vi "Simulation Interface.vi"(8 "error in (no error)":errorcluster, 11 "View Model":T1) -> (0 "error out":errorcluster, 3 "View Model":T1)   [LabVIEW 2017]
doc: "Main VI used to validate the CarWash controller logic and algorithms."
uses:
  Model/Controls/View Model.ctl
  Model/Controls/Shared Model.ctl
  Error Handler/Controls/Error Model.ctl
  Error Handler/Controls/Error Message.ctl
  Error Handler/Controls/Error Type.ctl
  Configuration/Controls/Config Model.ctl
  Configuration/Controls/Config DB Message.ctl
  Configuration/Controls/Config DB Command.ctl
  Configuration/Controls/Config DB Overhead.ctl
  Configuration/Controls/Config DB Record1.ctl
  Configuration/Controls/Config DB Record2.ctl
  Controller/Controls/Controller Wash Step.ctl
  Views/Vehicle Position Simulation View/Controls/Vehicle - Position.ctl
  Controller/Controls/Controller Model.ctl
  Controller/Controls/Controller Overhead.ctl
  Controller/Controls/Controller State.ctl
  Model/Controls/Interface.ctl
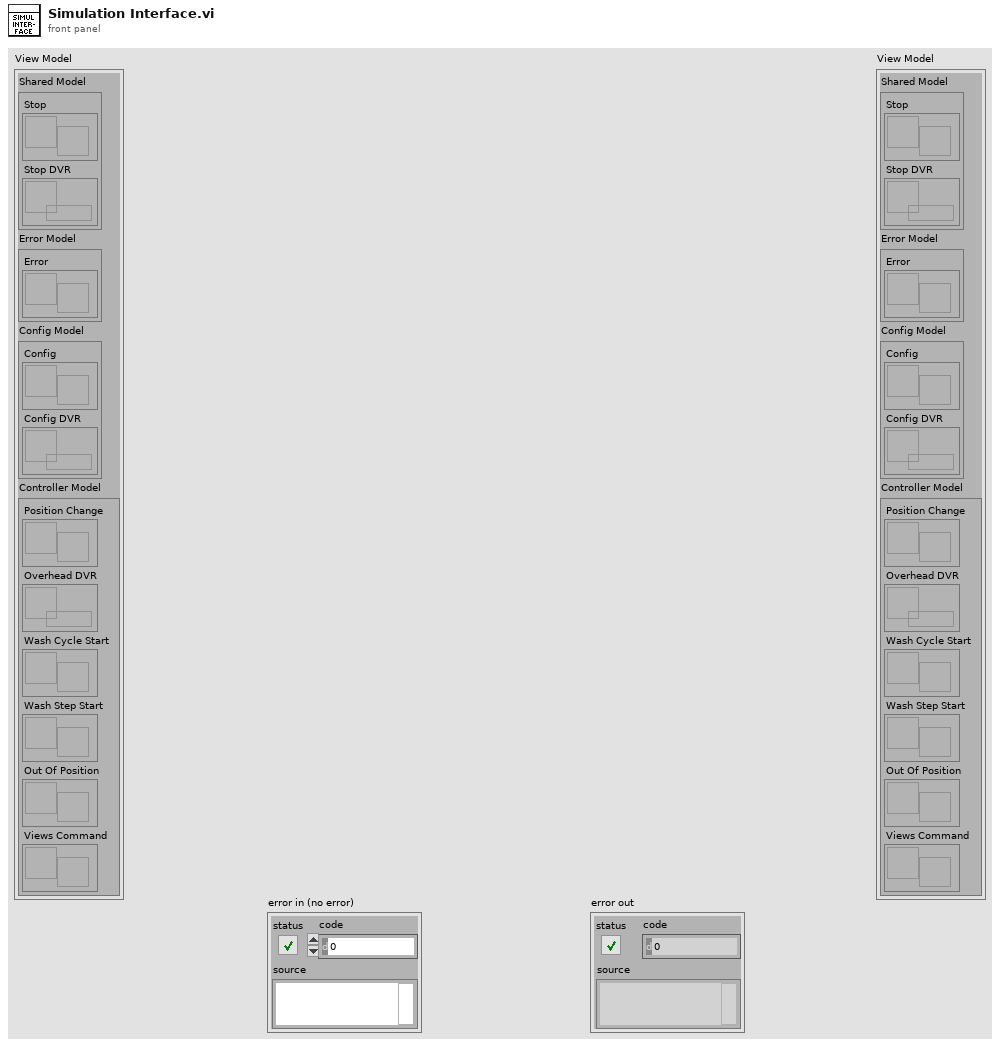
[diagram p1: front panel]
types:
  T1 = typedef "View Model.ctl" = cluster{"Shared Model":T2, "Error Model":T3, "Config Model":T4, "Controller Model":T5}
  T2 = typedef "Shared Model.ctl" = cluster{"Stop":refnum<user-event>, "Stop DVR":refnum<data-value>}
  T3 = typedef "Error Model.ctl" = cluster{"Error":refnum<user-event>}
  T4 = typedef "Config Model.ctl" = cluster{"Config":refnum<user-event>, "Config DVR":refnum<data-value>}
  T5 = typedef "Controller Model.ctl" = cluster{"Position Change":refnum<user-event>, "Overhead DVR":refnum<data-value>, "Wash Cycle Start":refnum<user-event>, "Wash Step Start":refnum<user-event>, "Out Of Position":refnum<user-event>, "Views Command":refnum<user-event>}
  T6 = typedef "Interface.ctl" = enum16{"Simulated", "Physical"}
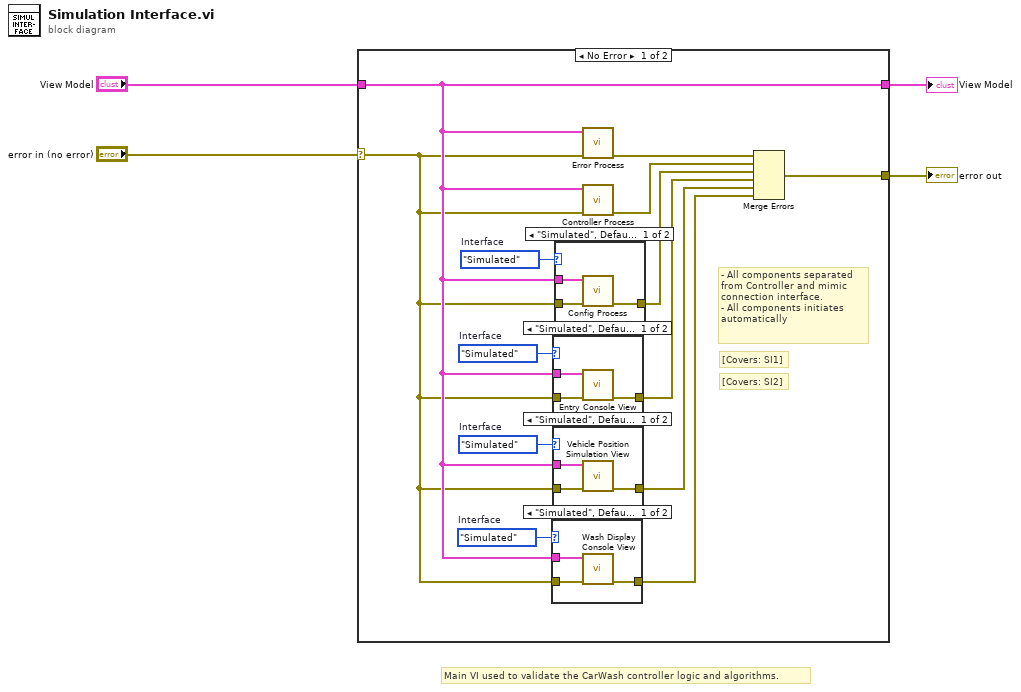
[diagram p0: block diagram]
diagram:
  # "Main VI used to validate the CarWash controller logic and algorithms."
  n1 = case shown="No Error" "error in (no error)" {
    selector: "error in (no error)" -> [w12 w34]
    tunnel: "View Model" -> [w13 w35]
    tunnel: [w5 w34] -> w2
    tunnel: [w13 w35] -> w1
    frame No Error {
      w14 = Interface."Simulated"  # Interface
      w15 = Interface."Simulated"  # Interface
      w16 = Interface."Simulated"  # Interface
      w17 = Interface."Simulated"  # Interface
      # "[Covers: SI2]"
      # "[Covers: SI1]"
      # "- All components separated\nfrom Controller and mimic\nconnection interface.\n- All components initiates \nautomatically"
      n2 = case shown="\"Simulated\", Default" w14 {
        tunnel: w12 -> [w19 w21]
        tunnel: [w20 w21] -> w6
        tunnel: w13 -> [w18 _]
        frame "Simulated", Default {
          n3 = call "Wash Display Console View.vi"("error in (no error)"=w19, "View Model"=w18) -> ("error out"=w20:errorcluster)  [unwired: 9 in]
        }
        frame "Physical" {
        }
      }
      n4 = case shown="\"Simulated\", Default" w16 {
        tunnel: w12 -> [w28 w29]
        tunnel: [w27 w29] -> w8
        tunnel: w13 -> [w26 _]
        frame "Simulated", Default {
          n5 = call "Entry Console View.vi"("error in (no error)"=w28, "View Model"=w26) -> ("error out"=w27:errorcluster)  [unwired: 9 in]
        }
        frame "Physical" {
        }
      }
      n6 = case shown="\"Simulated\", Default" w15 {
        tunnel: w12 -> [w23 w25]
        tunnel: [w24 w25] -> w7
        tunnel: w13 -> [w22 _]
        frame "Simulated", Default {
          n7 = call "Vehicle Position Simulation View.vi"("error in (no error)"=w23, "View Model"=w22) -> ("error out"=w24:errorcluster)  [unwired: 9 in]
        }
        frame "Physical" {
        }
      }
      n8 = case shown="\"Simulated\", Default" w17 {
        tunnel: w13 -> [w32 _]
        tunnel: w12 -> [w31 w33]
        tunnel: [w30 w33] -> w9
        frame "Simulated", Default {
          n9 = call "Config Process.vi"("error in (no error)"=w31, "View Model"=w32) -> ("error out"=w30:errorcluster)  [unwired: 9 in]
        }
        frame "Physical" {
        }
      }
      n10 = call "Error Process.vi"("error in (no error)"=w12, "View Model"=w13) -> ("error out"=w11:errorcluster)  [unwired: 9 in]
      n11 = call "Controller Process.vi"("error in (no error)"=w12, "View Model"=w13) -> ("error out"=w10:errorcluster)  [unwired: 9 in]
      n12 = Merge Errors(w11, w10, w9, w8, w7, w6) -> (w5:errorcluster)
    }
    frame Error {
    }
  }
  "View Model" <- w1
  "error out" <- w2
